vi "calculator(SubVI).vi"(11 "Numeric 11":i32) -> (3 "Numeric 10":i32)   [LabVIEW 2015]
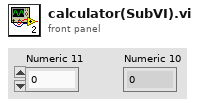
[diagram p1: front panel]
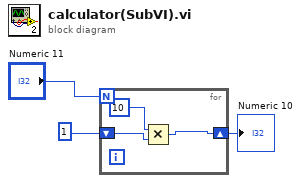
[diagram p0: block diagram]
diagram:
  n1 = for {
    N: "Numeric 11" -> [_]
    shift-right: [w5] -> w1
    shift-left: 1 -> [w6]
    n2 = Multiply(x=10, y=w6) -> (x*y=w5:i32)
  }
  "Numeric 10" <- w1
